vi "Log Viewer.vi"() -> ()   [LabVIEW 2015]
uses:
  <vilib>/Utility/miscctls.llb/LVRowAndColumnUnsignedTypeDef.ctl
panel:
  in  "Log Table":string[][](table)
  in  "clear":bool
  in  "stop":bool
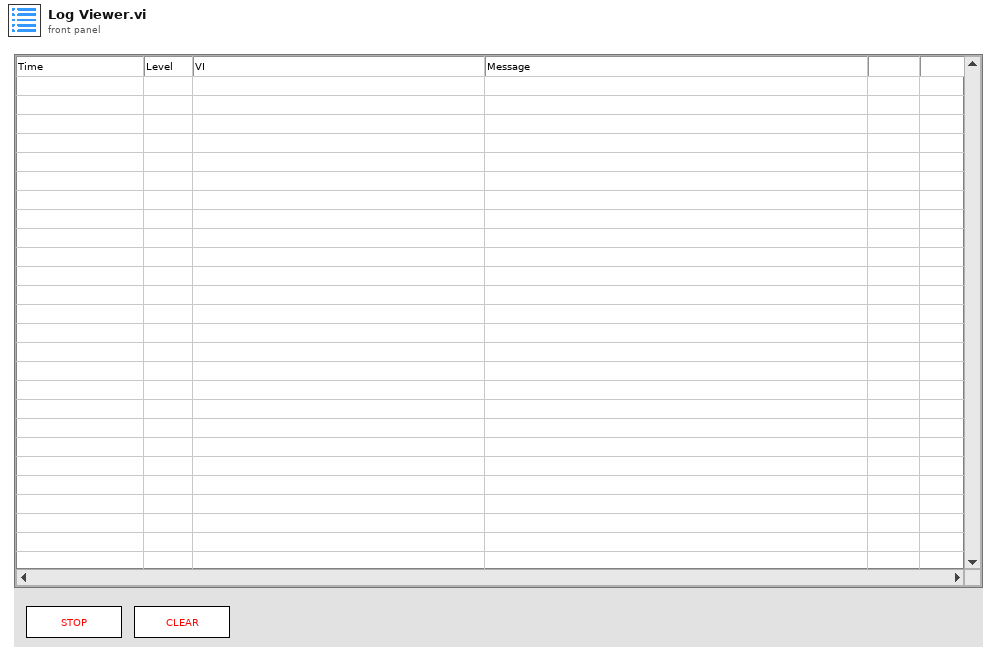
[diagram p1: front panel]
types:
  T1 = typedef "LVRowAndColumnUnsignedTypeDef.ctl" = cluster{"Row":u32, "Column":u32}
  T2 = cluster{"Log Level":enum16{"INFO", "DEBUG", "WARN", "ERROR"}, "Time Stamp":timestamp, "Call Chain":string[], "Message":string}
  T3 = enum32{"Invalid", "Standard", "Closed", "Hidden", "Minimized", "Maximized"}
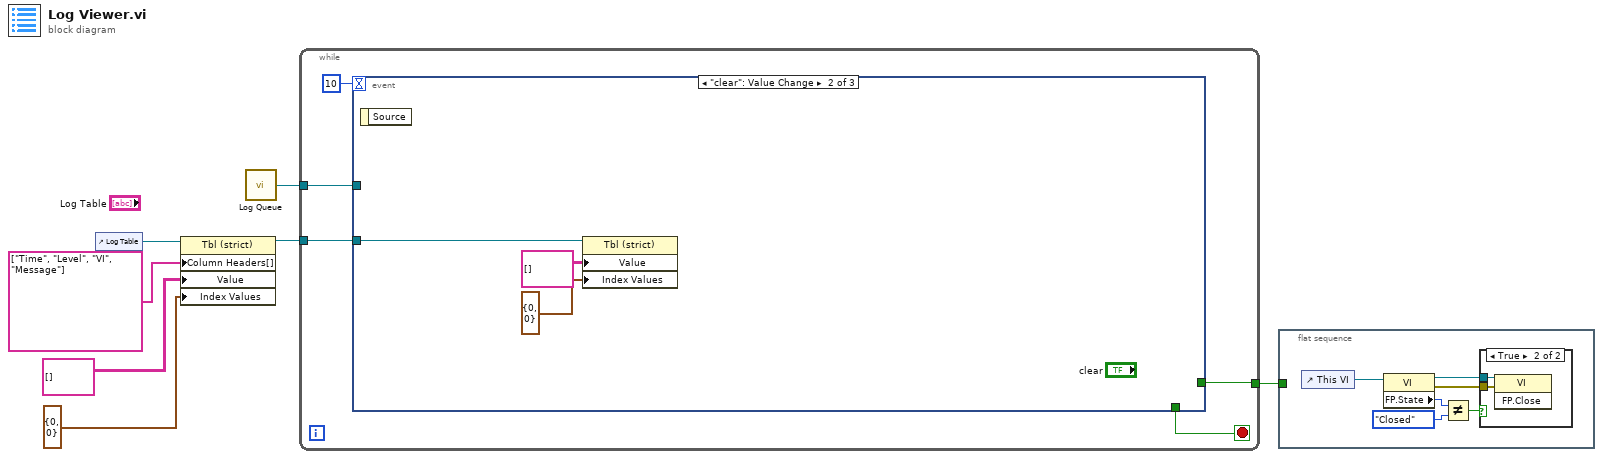
[diagram p0: block diagram]
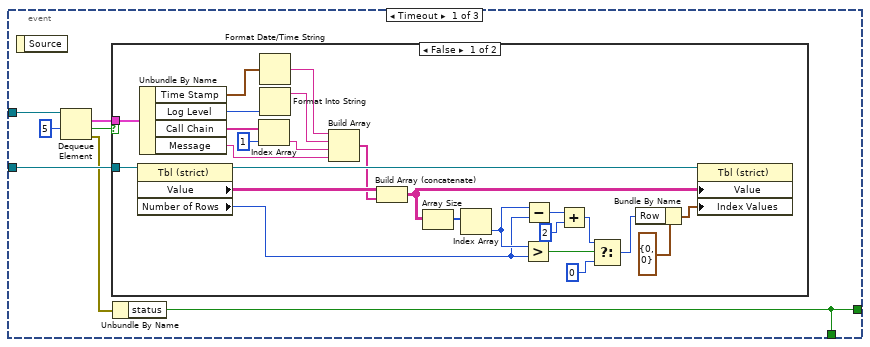
[diagram p3: hidden frame]
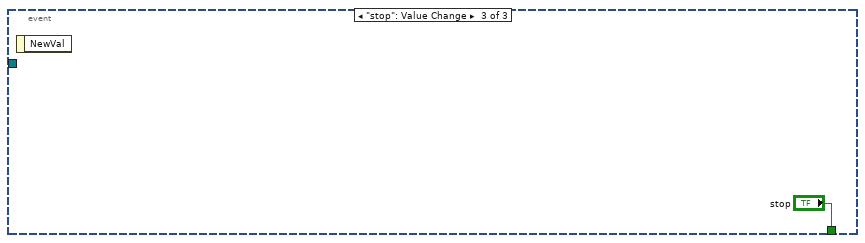
[diagram p5: hidden frame]
diagram:
  n1 = control-ref of="Log Table"() -> (w6:refnum<vi>)
  n2 = property class="Tbl (strict)"(reference=w6, "Column Headers[]"=string[] ["Time", "Level", "VI", "Message"] ("Column Header Strings[]"), "Value"=string[][] [], "Index Values"=T1 {"Row"=0, "Column"=0}) -> (reference out=w3:refnum<vi>)  [unwired: 1 in, 1 out]
  n3 = call "Log Queue.vi"() -> ("Log Queue"=w7:refnum<queue>)  [unwired: 5 in]
  n4 = while {
    tunnel: w7 -> [w11]
    tunnel: w3 -> [w9]
    tunnel: [w8] -> w1
    stop <- w10 stop-if-true
    n5 = event shown="[1] \"clear\": Value Change" {
      selector: _ -> [_ _ _]
      dyn-events: _ -> [_ _ _]
      timeout: 10 -> [_ _ _]
      tunnel: w11 -> [w19 _ _]
      tunnel: [w13 _ "stop"] -> w10
      tunnel: w9 -> [w15 w47 _]
      tunnel: [w13 _ _] -> w8
      event Timeout {
        n6 = event-data() -> ()  [unwired: 1 in, 1 out]
        n7 = Dequeue Element(queue=w19, timeout in ms (-1)=5) -> (element=w16:T2, timed out?=w17:bool, error out=w14:errorcluster)  [unwired: 1 in, 1 out]
        n8 = case shown="False" w17 {
          tunnel: w16 -> [w42 _]
          tunnel: w15 -> [w44 _]
          frame False {
            n9 = property class="Tbl (strict)"(reference=w44) -> (reference out=w43:refnum<vi>, "Value"=w33:string[][], "Number of Rows"=w24:u32)  [unwired: 1 in, 1 out]
            n10 = Unbundle By Name(w42) -> ("Time Stamp"=w41:timestamp, "Log Level"=w40:enum16{"INFO", "DEBUG", "WARN", "ERROR"}, "Call Chain"=w39:string[], "Message"=w37:string)
            n11 = Index Array(array=w39, index=1) -> (element=w36:string)
            n12 = Format Date/Time String(seconds (now)=w41) -> (date/time string=w34:string)  [unwired: 2 in]
            n13 = Format Into String(w40) -> (resulting string=w35:string)  [unwired: 3 in, 1 out]
            n14 = Build Array(w34, w35, w36, w37) -> (w32:string[])
            n15 = Build Array (concatenate)(w33, w32) -> (w31:string[][])
            n16 = Array Size(array=w31) -> (size(s)=w28:i32[])
            n17 = Index Array(array=w28) -> (element=w25:i32)  [unwired: 1 in]
            n18 = Greater?(x=w25, y=w24) -> (0:w27:bool)
            n19 = Subtract(x=w25, y=w24) -> (x-y=w22:u32)
            n20 = Add(x=w22, y=u32 2) -> (x+y=w21:u32)
            n21 = Select(t=w21, s=w27, f=u32 0) -> (s? t:f=w23:u32)
            n22 = Bundle By Name(cluster=T1 {"Row"=0, "Column"=0} ("Index Values"), "Row"=w23) -> (w29:T1)
            n23 = property class="Tbl (strict)"(reference=w43, "Value"=w31, "Index Values"=w29) -> ()  [unwired: 1 in, 2 out]
          }
          frame True {
          }
        }
        n24 = Unbundle By Name(w14) -> ("status"=w13:bool)
      }
      event "clear": Value Change {
        n25 = event-data() -> ()  [unwired: 1 in, 1 out]
        n26 = property class="Tbl (strict)"(reference=w47, "Value"=string[][] [], "Index Values"=T1 {"Row"=0, "Column"=0}) -> ()  [unwired: 1 in, 2 out]
      }
      event "stop": Value Change {
        n27 = event-data() -> ()  [unwired: 1 in, 1 out]
      }
    }
  }
  n28 = flat-sequence {
    tunnel: w1 -> [_]
    frame #0 {
      n29 = control-ref of="This VI"() -> (w54:refnum<vi>)
      n30 = property class="VI"(reference=w54) -> (reference out=w51:refnum<vi>, error out=w50:errorcluster, "FP.State"=w53:T3)  [unwired: 1 in]
      n31 = Not Equal?(x=w53, y=T3."Closed" ("Front Panel Window:State")) -> (x != y?=w49:bool)
      n32 = case shown="True" w49 {
        tunnel: w51 -> [_ w56]
        tunnel: w50 -> [_ w55]
        frame False {
        }
        frame True {
          n33 = invoke class="VI" method="FP.Close"(reference=w56, error in=w55) -> ()  [unwired: 1 in, 3 out]
        }
      }
    }
  }
